vi "_Calibrate DAC 2.vi"(1 "Table Type":T1, 2 "Current Mass":i32) -> (0 "DAC":u32)   [LabVIEW 2012]
uses:
  Type/_Table Type.ctl
  <vilib>/rvi/DataTransferAndStorage/Container/Common/niFpgaContainerGetUniqueNameForEmu.vi
  <vilib>/rvi/Memory/Memory_Emulation/niFpgaMemoryEmulationCacheClearOnFirstRun.vi
  <vilib>/rvi/Memory/Memory_Emulation/nirvimemoryEmulationManagerCache_MakeExclusive.vi
  <vilib>/rvi/Memory/Memory_Emulation/niFpgaMemoryEmulationValidateCache.vi
  <vilib>/rvi/Memory/Memory_Emulation/nirvimemoryEmulationManagerCache_ReleaseExclusive.vi
  <vilib>/rvi/Memory/Memory_Emulation/nirvimemoryEmulationManagerCache_InsertValue.vi
  <vilib>/Utility/error.llb/Clear Errors.vi
  <vilib>/rvi/Memory/Memory_Emulation/nirvimemoryEmulationManagerCache_GetValue.vi
  <vilib>/rvi/DataTransferAndStorage/Container/XNode/niFpgaContainer.xnode
  <vilib>/rvi/Memory/Memory_Emulation/nirvimemoryEmulation.vi
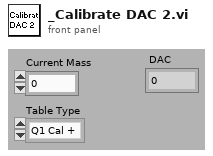
[diagram p1: front panel]
types:
  T1 = typedef "_Table Type.ctl" = enum8{"Q1 Cal +", "Q2 Cal +", "Q1 Cal -", "Q2 Cal -", "Q1 Res Hi +", "Q2 Res Hi +", "Q1 Res Med +", "Q2 Res Med +", "Q1 Res Lo +", "Q2 Res Lo +", "Q1 Res Hi -", "Q2 Res Hi -", "Q1 Res Med -", "Q2 Res Med -", "Q1 Res Lo -", "Q2 Res Lo -"}
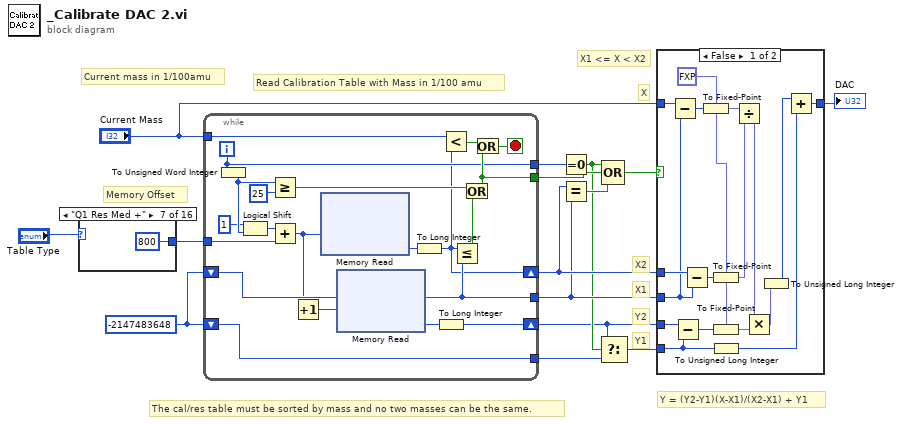
[diagram p0: block diagram]
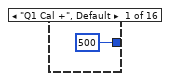
[diagram p2: hidden frame]
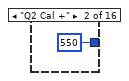
[diagram p3: hidden frame]
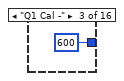
[diagram p4: hidden frame]
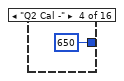
[diagram p5: hidden frame]
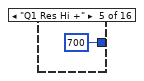
[diagram p6: hidden frame]
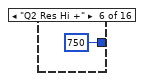
[diagram p7: hidden frame]
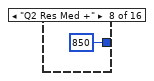
[diagram p8: hidden frame]
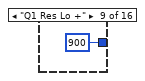
[diagram p9: hidden frame]
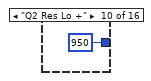
[diagram p10: hidden frame]
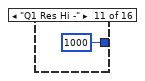
[diagram p11: hidden frame]
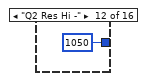
[diagram p12: hidden frame]
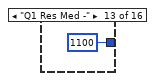
[diagram p13: hidden frame]
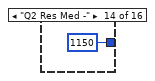
[diagram p14: hidden frame]
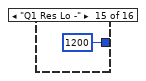
[diagram p15: hidden frame]
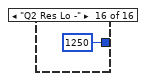
[diagram p16: hidden frame]
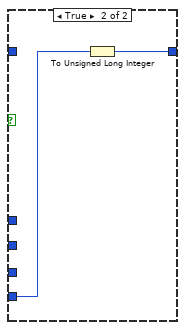
[diagram p17: hidden frame]
diagram:
  w13 = -2147483648 ("Data")
  # "X1 <= X < X2"
  # "Y = (Y2-Y1)(X-X1)/(X2-X1) + Y1"
  # "The cal/res table must be sorted by mass and no two masses can be the same."
  # "Memory Offset"
  # "Current mass in 1/100amu"
  # "Read Calibration Table with Mass in 1/100 amu"
  # "X"
  # "Y2"
  # "Y1"
  # "X2"
  # "X1"
  n1 = case shown="\"Q1 Res Med +\"" "Table Type" {
    tunnel: [u16 500 ("Addr Offset") u16 550 ("Addr Offset") u16 600 ("Addr Offset") u16 650 ("Addr Offset") u16 700 ("Addr Offset") u16 750 ("Addr Offset") u16 800 ("Addr Offset") u16 850 ("Addr Offset") u16 900 ("Addr Offset") u16 950 ("Addr Offset") u16 1000 ("Addr Offset") u16 1050 ("Addr Offset") u16 1100 ("Addr Offset") u16 1150 ("Addr Offset") u16 1200 ("Addr Offset") u16 1250 ("Addr Offset")] -> w3
    frame "Q1 Cal +", Default {
    }
    frame "Q2 Cal +" {
    }
    frame "Q1 Cal -" {
    }
    frame "Q2 Cal -" {
    }
    frame "Q1 Res Hi +" {
    }
    frame "Q2 Res Hi +" {
    }
    frame "Q1 Res Med +" {
    }
    frame "Q2 Res Med +" {
    }
    frame "Q1 Res Lo +" {
    }
    frame "Q2 Res Lo +" {
    }
    frame "Q1 Res Hi -" {
    }
    frame "Q2 Res Hi -" {
    }
    frame "Q1 Res Med -" {
    }
    frame "Q2 Res Med -" {
    }
    frame "Q1 Res Lo -" {
    }
    frame "Q2 Res Lo -" {
    }
  }
  n2 = while {
    tunnel: "Current Mass" -> [w50]
    tunnel: w3 -> [w49]
    shift-right: [w40] -> w15
    shift-left: w13 -> [w42]
    shift-right: [w39] -> w7
    shift-left: w13 -> [w41]
    tunnel: [w41] -> w5
    tunnel: [w42] -> w14
    tunnel: [w44] -> w11
    tunnel: [w43] -> w12
    i -> [w43]
    stop <- w45 stop-if-true
    n3 = To Unsigned Word Integer(number=w43) -> (unsigned 16bit integer=w38:u16)
    n4 = Logical Shift(y=u16 1, x=w38) -> (x << y=w37:u16)
    n5 = Greater Or Equal?(x=w38, y=u16 25) -> (x >= y?=w47:bool)
    n6 = Add(x=w37, y=w49) -> (x+y=w35:u16)
    n7 = Increment(x=w35) -> (x+1=w32:u16)
    n8 = xnode "Memory Read"("Address"=w35) -> ("Data"=w34:u32)  [unwired: 1 in, 1 out]
    n9 = xnode "Memory Read"("Address"=w32) -> ("Data"=w33:u32)  [unwired: 1 in, 1 out]
    n10 = To Long Integer(number=w34) -> (32bit integer=w40:i32)
    n11 = To Long Integer(number=w33) -> (32bit integer=w39:i32)
    n12 = Less?(x=w50, y=w40) -> (x < y?=w46:bool)
    n13 = Less Or Equal?(x=w40, y=w42) -> (x <= y?=w48:bool)
    n14 = Or(x=w47, y=w48) -> (x .or. y?=w44:bool)
    n15 = Or(x=w46, y=w44) -> (x .or. y?=w45:bool)
  }
  n16 = Equal To 0?(x=w12) -> (x = 0?=w8:bool)
  n17 = Equal?(x=w15, y=w14) -> (x = y?=w10:bool)
  n18 = Select(t=w7, s=w8, f=w5) -> (s? t:f=w6:i32)
  n19 = Compound Arithmetic op=OR(w8, w11, w10) -> (w9:bool)
  n20 = case shown="False" w9 {
    tunnel: "Current Mass" -> [w68 _]
    tunnel: w7 -> [w61 _]
    tunnel: w6 -> [w55 w70]
    tunnel: [w53 w69] -> w1
    tunnel: w14 -> [w66 _]
    tunnel: w15 -> [w67 _]
    frame False {
      w57 = fxp<+,32,22> 0.0
      n21 = Subtract(x=w68, y=w66) -> (x-y=w65:i32)
      n22 = Subtract(x=w61, y=w55) -> (x-y=w60:i32)
      n23 = Subtract(x=w67, y=w66) -> (x-y=w64:i32)
      n24 = To Fixed-Point(fixed-point type=w57, number=w65) -> (fixed-point=w63:fxp<+,32,22>)
      n25 = To Fixed-Point(fixed-point type=w57, number=w64) -> (fixed-point=w62:fxp<+,32,22>)
      n26 = To Fixed-Point(fixed-point type=w57, number=w60) -> (fixed-point=w58:fxp<+,32,22>)
      n27 = To Unsigned Long Integer(number=w55) -> (unsigned 32bit integer=w52:u32)
      n28 = Divide(x=w63, y=w62) -> (x/y=w59:fxp<+,32,0>)
      n29 = Multiply(x=w59, y=w58) -> (x*y=w56:fxp<+,32,32>)
      n30 = To Unsigned Long Integer(number=w56) -> (unsigned 32bit integer=w54:u32)
      n31 = Add(x=w54, y=w52) -> (x+y=w53:u32)
    }
    frame True {
      n32 = To Unsigned Long Integer(number=w70) -> (unsigned 32bit integer=w69:u32)
    }
  }
  "DAC" <- w1
